vi "SetElementDecode.vi"(10 "Payload":string) -> (2 "RequestIDRec":T1, 3 "number of items":u8)   [LabVIEW 2009]
uses:
  Support Files/RequestIDRec.ctl
  Support Files/ElementRec.ctl
  Support Files/LocalWaypointRec.ctl
panel:
  out "Offset":string
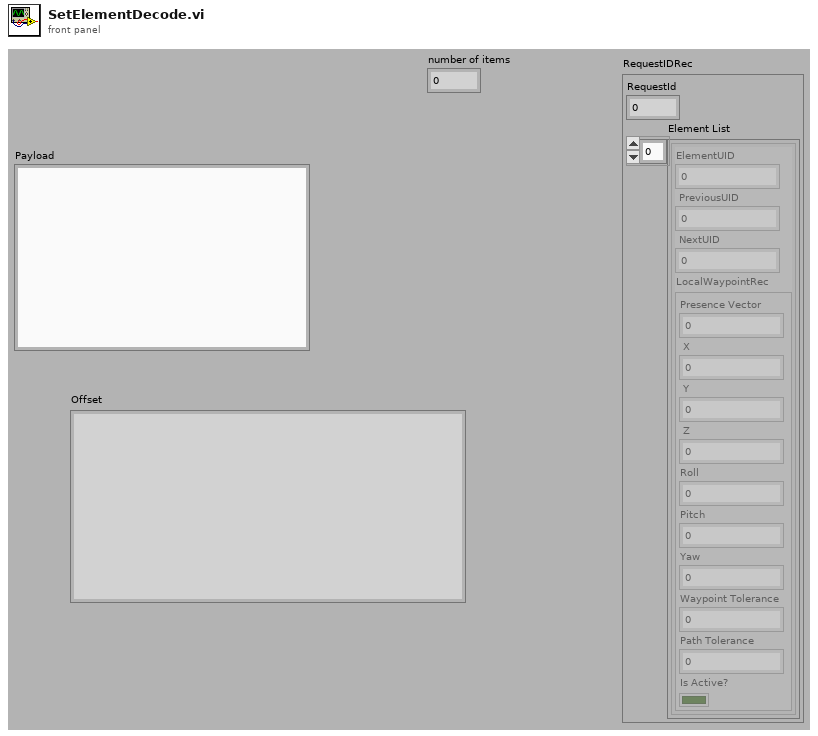
[diagram p1: front panel]
types:
  T1 = typedef "RequestIDRec.ctl" = cluster{"RequestId":u8, "Element List":T2[]}
  T2 = typedef "ElementRec.ctl" = cluster{"ElementUID":u16, " PreviousUID":u16, " NextUID":u16, "LocalWaypointRec":T3}
  T3 = typedef "LocalWaypointRec.ctl" = cluster{"Presence Vector":u8, " X":dbl, " Y":dbl, " Z":dbl, "Roll":dbl, "Pitch":dbl, "Yaw":dbl, "Waypoint Tolerance":dbl, "Path Tolerance":dbl, "Is Active?":bool}
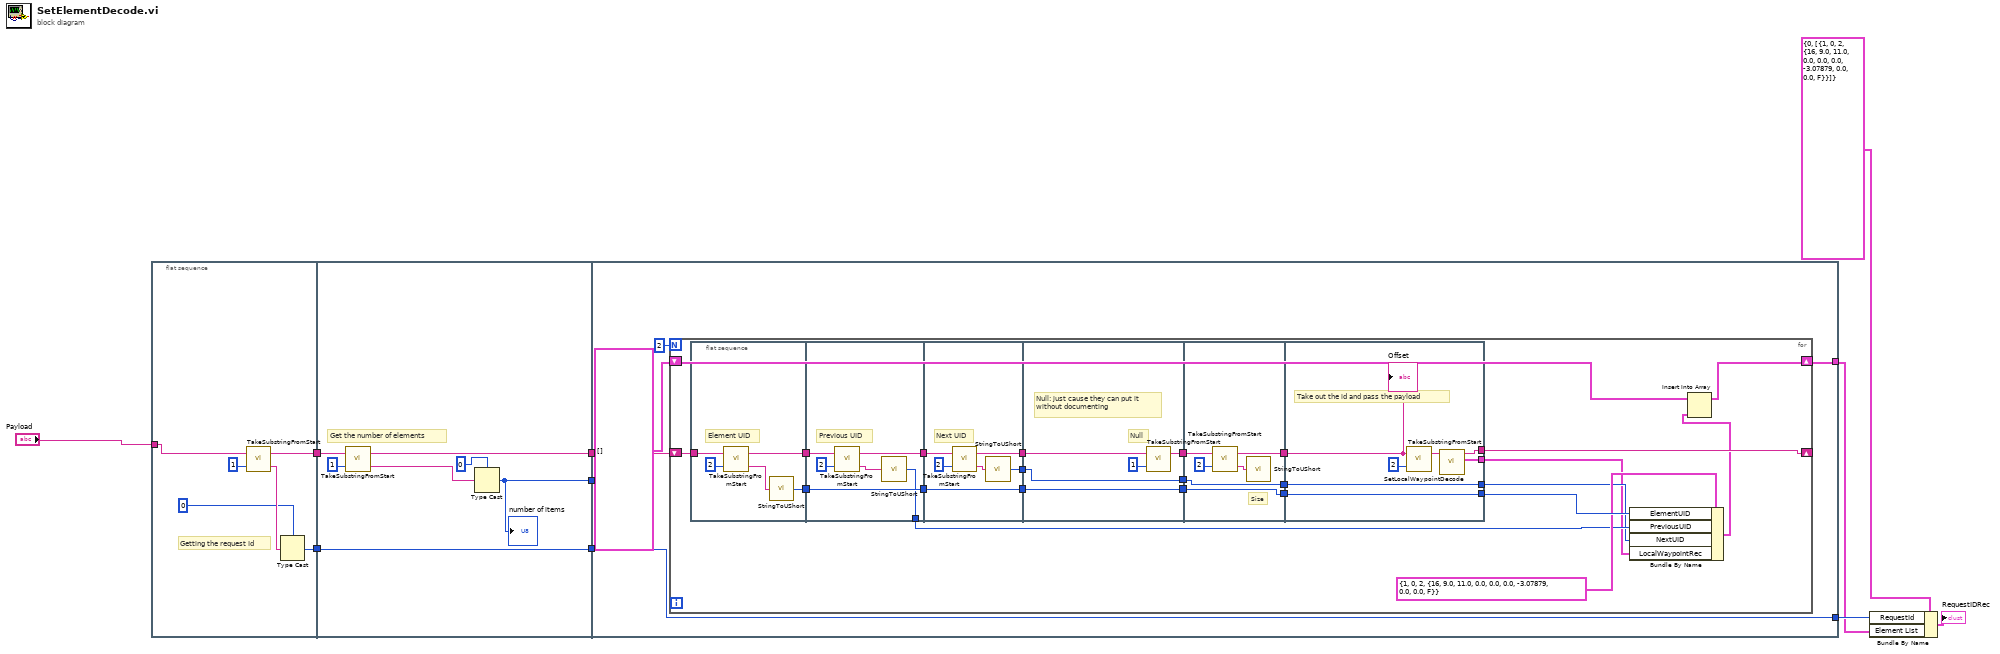
[diagram p0: block diagram]
diagram:
  n1 = flat-sequence {
    tunnel: [w15] -> w10
    tunnel: [w12] -> w9
    tunnel: "Payload" -> [w11]
    tunnel: w10 -> [w22]
    tunnel: w9 -> [w21]
    tunnel: [w21] -> w6
    tunnel: [w18] -> w5
    tunnel: [w17] -> w3
    tunnel: [w28] -> w8
    tunnel: w6 -> [w28]
    tunnel: w5 -> [_]
    tunnel: w3 -> [w27]
    tunnel: [w25] -> w2
    frame #0 {
      # "Getting the request Id"
      n2 = call "TakeSubstringFromStart.vi"("offset"=1, "string"=w11) -> ("string before offset"=w14:string, "string after offset"=w15:string)
      n3 = Type Cast(type=u8 0 ("offset"), x=w14) -> (*(type *) &x=w12:u8)
    }
    frame #1 {
      # "Get the number of elements"
      n4 = call "TakeSubstringFromStart.vi"("offset"=1, "string"=w22) -> ("string before offset"=w19:string, "string after offset"=w17:string)
      n5 = Type Cast(type=u8 0 ("offset"), x=w19) -> (*(type *) &x=w18:u8)
      "number of items" <- w18
    }
    frame #2 {
      n6 = for {
        N: 2 -> [_]
        shift-right: [w37] -> _
        shift-left: w27 -> [w29]
        shift-right: [w30] -> w25
        shift-left: T2[] [] -> [w32]
        n7 = flat-sequence {
          tunnel: w29 -> [w55]
          tunnel: [w53] -> w50
          tunnel: [w52] -> w49
          tunnel: w50 -> [w62]
          tunnel: w49 -> [w57]
          tunnel: [w62] -> w48
          tunnel: [w58] -> w47
          tunnel: [w59] -> w45
          tunnel: w48 -> [w68]
          tunnel: w47 -> [w65]
          tunnel: [w68] -> w43
          tunnel: [w64] -> w42
          tunnel: [w63] -> w41
          tunnel: w43 -> [w73]
          tunnel: w42 -> [w72]
          tunnel: w41 -> [w71]
          tunnel: [w73] -> w40
          tunnel: [w72] -> w39
          tunnel: [w69] -> w38
          tunnel: w40 -> [w79]
          tunnel: w39 -> [w78]
          tunnel: w38 -> [w75]
          tunnel: [w79] -> w36
          tunnel: [w78] -> w35
          tunnel: [w74] -> w34
          tunnel: [w83] -> w37
          tunnel: [w85] -> w44
          tunnel: [w86] -> w51
          tunnel: w36 -> [w86]
          tunnel: w35 -> [w85]
          tunnel: w34 -> [w80]
          tunnel: [w84] -> w33
          frame #0 {
            # "Element UID"
            n8 = call "TakeSubstringFromStart.vi"("offset"=2, "string"=w55) -> ("string before offset"=w54:string, "string after offset"=w52:string)
            n9 = call "StringToUShort.vi"("string"=w54) -> ("UShort"=w53:u16)
          }
          frame #1 {
            # "Previous UID"
            n10 = call "TakeSubstringFromStart.vi"("offset"=2, "string"=w57) -> ("string before offset"=w61:string, "string after offset"=w58:string)
            n11 = call "StringToUShort.vi"("string"=w61) -> ("UShort"=w59:u16)
          }
          frame #2 {
            # "Next UID"
            n12 = call "TakeSubstringFromStart.vi"("offset"=2, "string"=w65) -> ("string before offset"=w67:string, "string after offset"=w63:string)
            n13 = call "StringToUShort.vi"("string"=w67) -> ("UShort"=w64:u16)
          }
          frame #3 {
            # "Null: just cause they can put it\nwithout documenting"
            # "Null"
            n14 = call "TakeSubstringFromStart.vi"("offset"=1, "string"=w71) -> ("string after offset"=w69:string)  [unwired: 1 out]
          }
          frame #4 {
            # "Size"
            n15 = call "TakeSubstringFromStart.vi"("offset"=2, "string"=w75) -> ("string before offset"=w77:string, "string after offset"=w74:string)
            n16 = call "StringToUShort.vi"("string"=w77) -> ()  [unwired: 1 out]
          }
          frame #5 {
            # "Take out the id and pass the payload"
            n17 = call "TakeSubstringFromStart.vi"("offset"=2, "string"=w80) -> ("string after offset"=w81:string)  [unwired: 1 out]
            n18 = call "SetLocalWaypointDecode.vi"("Payload"=w81) -> ("LocalWaypointRec"=w84:T3, "string after offset"=w83:string)  [unwired: 9 in]
            "Offset" <- w80
          }
        }
        n19 = Bundle By Name(cluster=T2 {"ElementUID"=1, " PreviousUID"=0, " NextUID"=2, "LocalWaypointRec"={"Presence Vector"=16, " X"=9.0, " Y"=11.0, " Z"=0.0, "Roll"=0.0, "Pitch"=0.0, "Yaw"=-3.07879, "Waypoint Tolerance"=0.0, "Path Tolerance"=0.0, "Is Active?"=FALSE}} ("ElementRec"), "ElementUID"=w51, "PreviousUID"=w45, "NextUID"=w44, "LocalWaypointRec"=w33) -> (w31:T2)
        n20 = Insert Into Array(array=w32, new element=w31) -> (w30:T2[])  [unwired: 1 in]
      }
    }
  }
  n21 = Bundle By Name(cluster=T1 {"RequestId"=0, "Element List"=[{"ElementUID"=1, " PreviousUID"=0, " NextUID"=2, "LocalWaypointRec"={"Presence Vector"=16, " X"=9.0, " Y"=11.0, " Z"=0.0, "Roll"=0.0, "Pitch"=0.0, "Yaw"=-3.07879, "Waypoint Tolerance"=0.0, "Path Tolerance"=0.0, "Is Active?"=FALSE}}]} ("RequestIDRec"), "RequestId"=w8, "Element List"=w2) -> (→"RequestIDRec":T1)
